vi "Set Description.vi"(8 "error in (no error)":errorcluster, 10 "Description":string, 11 "PDO Mapping in":refnum<class "PDO Mapping.lvclass">) -> (0 "error out":errorcluster, 3 "PDO Mapping out":refnum<class "PDO Mapping.lvclass">)   [LabVIEW 2019, in "PDO Grid.lvlib" / "PDO Mapping.lvclass"]
uses:
  PDO Mapping.lvclass
  PDO Mapping.lvclass/PDO Mapping.ctl
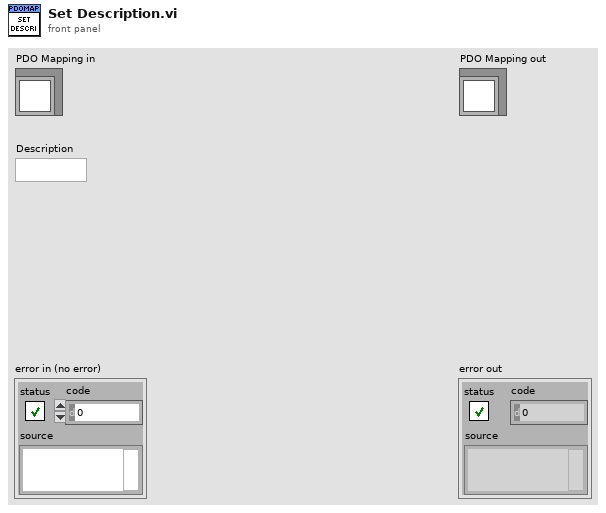
[diagram p1: front panel]
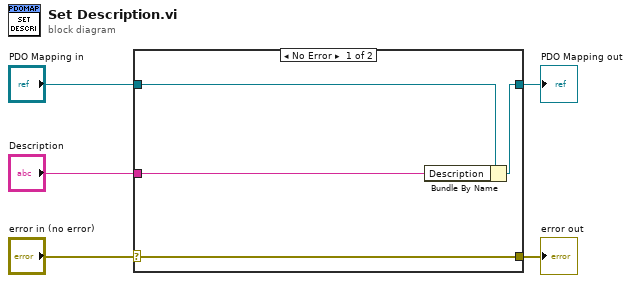
[diagram p0: block diagram]
diagram:
  n1 = case shown="No Error" "error in (no error)" {
    selector: "error in (no error)" -> [w9 w10]
    tunnel: [w9 w10] -> w4
    tunnel: [w7 w11] -> w2
    tunnel: "PDO Mapping in" -> [w8 w11]
    tunnel: "Description" -> [w6 _]
    frame No Error {
      n2 = Bundle By Name(cluster=w8, "Description"=w6) -> (w7:refnum<class "PDO Mapping.lvclass">)
    }
    frame Error {
    }
  }
  "error out" <- w4
  "PDO Mapping out" <- w2
